vi "Game Mech.vi"() -> ()   [LabVIEW 2014]
uses:
  <vilib>/Rock Robotics/WPI/Solenoid/WPI_SolenoidValue.ctl
  <vilib>/Rock Robotics/WPI/Joystick/WPI_JoystickGetSetRefNum.vi
  <vilib>/Rock Robotics/Network Tables/SD Write Boolean Array.vi
  <vilib>/Rock Robotics/Network Tables/SD Write Numeric Array.vi
  <vilib>/Rock Robotics/WPI/Solenoid/WPI_SolenoidSetEnum.vi
  <vilib>/Rock Robotics/Network Tables/SD Write Number.vi
  <vilib>/addons/control/pid/NI_PID_pid.lvlib
  <vilib>/addons/control/pid/pid.llb/PID (DBL).vi
panel:
  in  "Controlling Mech":enum16{"Arm", "Left 2CAN", "Right 2CAN"}(ring)
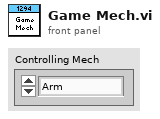
[diagram p1: front panel]
types:
  T1 = typedef "WPI_JoystickDevRef.ctl" = cluster{"Device":T2}
  T2 = typedef "WPI_JoystickDeviceEnum.ctl" = enum16{"USB 0", "USB 1", "USB 2", "USB 3", "USB 4", "USB 5"}
  T3 = cluster{"proportional gain (Kc)":dbl, "integral time (Ti, min)":dbl, "derivative time (Td, min)":dbl}
  T4 = typedef "WPI_PotentiometerDevRef.ctl" = cluster{"DevStatus":errorcluster, "Controller":T5, "Analog Channel":T6, "Invert Output":bool}
  T5 = typedef "FPGA_TypedefAnalogModule.ctl" = enum16{"Controller 1"}
  T6 = typedef "FPGA_AIChannel.ctl" = enum8{"AI 0", "AI 1", "AI 2", "AI 3", "AI MXP 0", "AI MXP 1", "AI MXP 2", "AI MXP 3", "Invalid"}
  T7 = typedef "WPI_SolenoidValue.ctl" = enum16{"Off", "On", "Forward", "Reverse"}
  T8 = typedef "WPI_SolenoidDevRef.ctl" = cluster{"DevStatus":errorcluster, "Pneumatics Control Module":u8, "Forward Solenoid Channel":T9, "Reverse Solenoid Channel":T9}
  T9 = typedef "WPI_SolenoidChannel.ctl" = enum8{"Solenoid 0", "Solenoid 1", "Solenoid 2", "Solenoid 3", "Solenoid 4", "Solenoid 5", "Solenoid 6", "Solenoid 7", "Invalid"}
  T10 = typedef "WPI_MotorControlDeviceRef.ctl" = cluster{"DeviceStatus":errorcluster, "Type":T11, "PWM":cluster{"Controller":T12, "PWM Channel":T13, "DeadBand":T14}, "CAN":cluster{"Device Number":u8, "Control Mode":T15, "Semaphore":T16, "Max Vout":dbl, "TalonSRX Control Mode":T17}, "Invert":bool, "TransformRef":T18, "InvTransformRef":T18}
  T11 = typedef "WPI_MotorControlType.ctl" = enum16{"PWM", "CAN", "CANTalonSRX"}
  T12 = typedef "FPGA_TypedefDigitalModule.ctl" = enum16{"Controller 1"}
  T13 = typedef "FPGA_DIOPWMChannel.ctl" = enum8{"PWM 0", "PWM 1", "PWM 2", "PWM 3", "PWM 4", "PWM 5", "PWM 6", "PWM 7", "PWM 8", "PWM 9", "PWM MXP 0", "PWM MXP 1", "PWM MXP 2", "PWM MXP 3", "PWM MXP 4", "PWM MXP 5", "PWM MXP 6", "PWM MXP 7", "PWM MXP 8", "PWM MXP 9", "Invalid"}
  T14 = typedef "WPI_PWMDeadband.ctl" = cluster{"Name":string, "maxPositivePwm":i32, "minPositivePwm":i32, "centerPwm":i32, "maxNegativePwm":i32, "minNegativePwm":i32, "angularRange":u16}
  T15 = typedef "WPI_CANJaguar_ControlMode.ctl" = enum8{"Percent VBus", "Current", "Speed", "Position", "Voltage"}
  T16 = typedef "Semaphore RefNum" = refnum<k1>
  T17 = typedef "WPI_CANTalonSRX_APIControlMode.ctl" = enum8{"Percent VBus", "Speed", "Position", "Slave", "Unchanged / Invalid"}
  T18 = typedef "WPI_PWMTransform_ConPane.ctl" = refnum<vi>
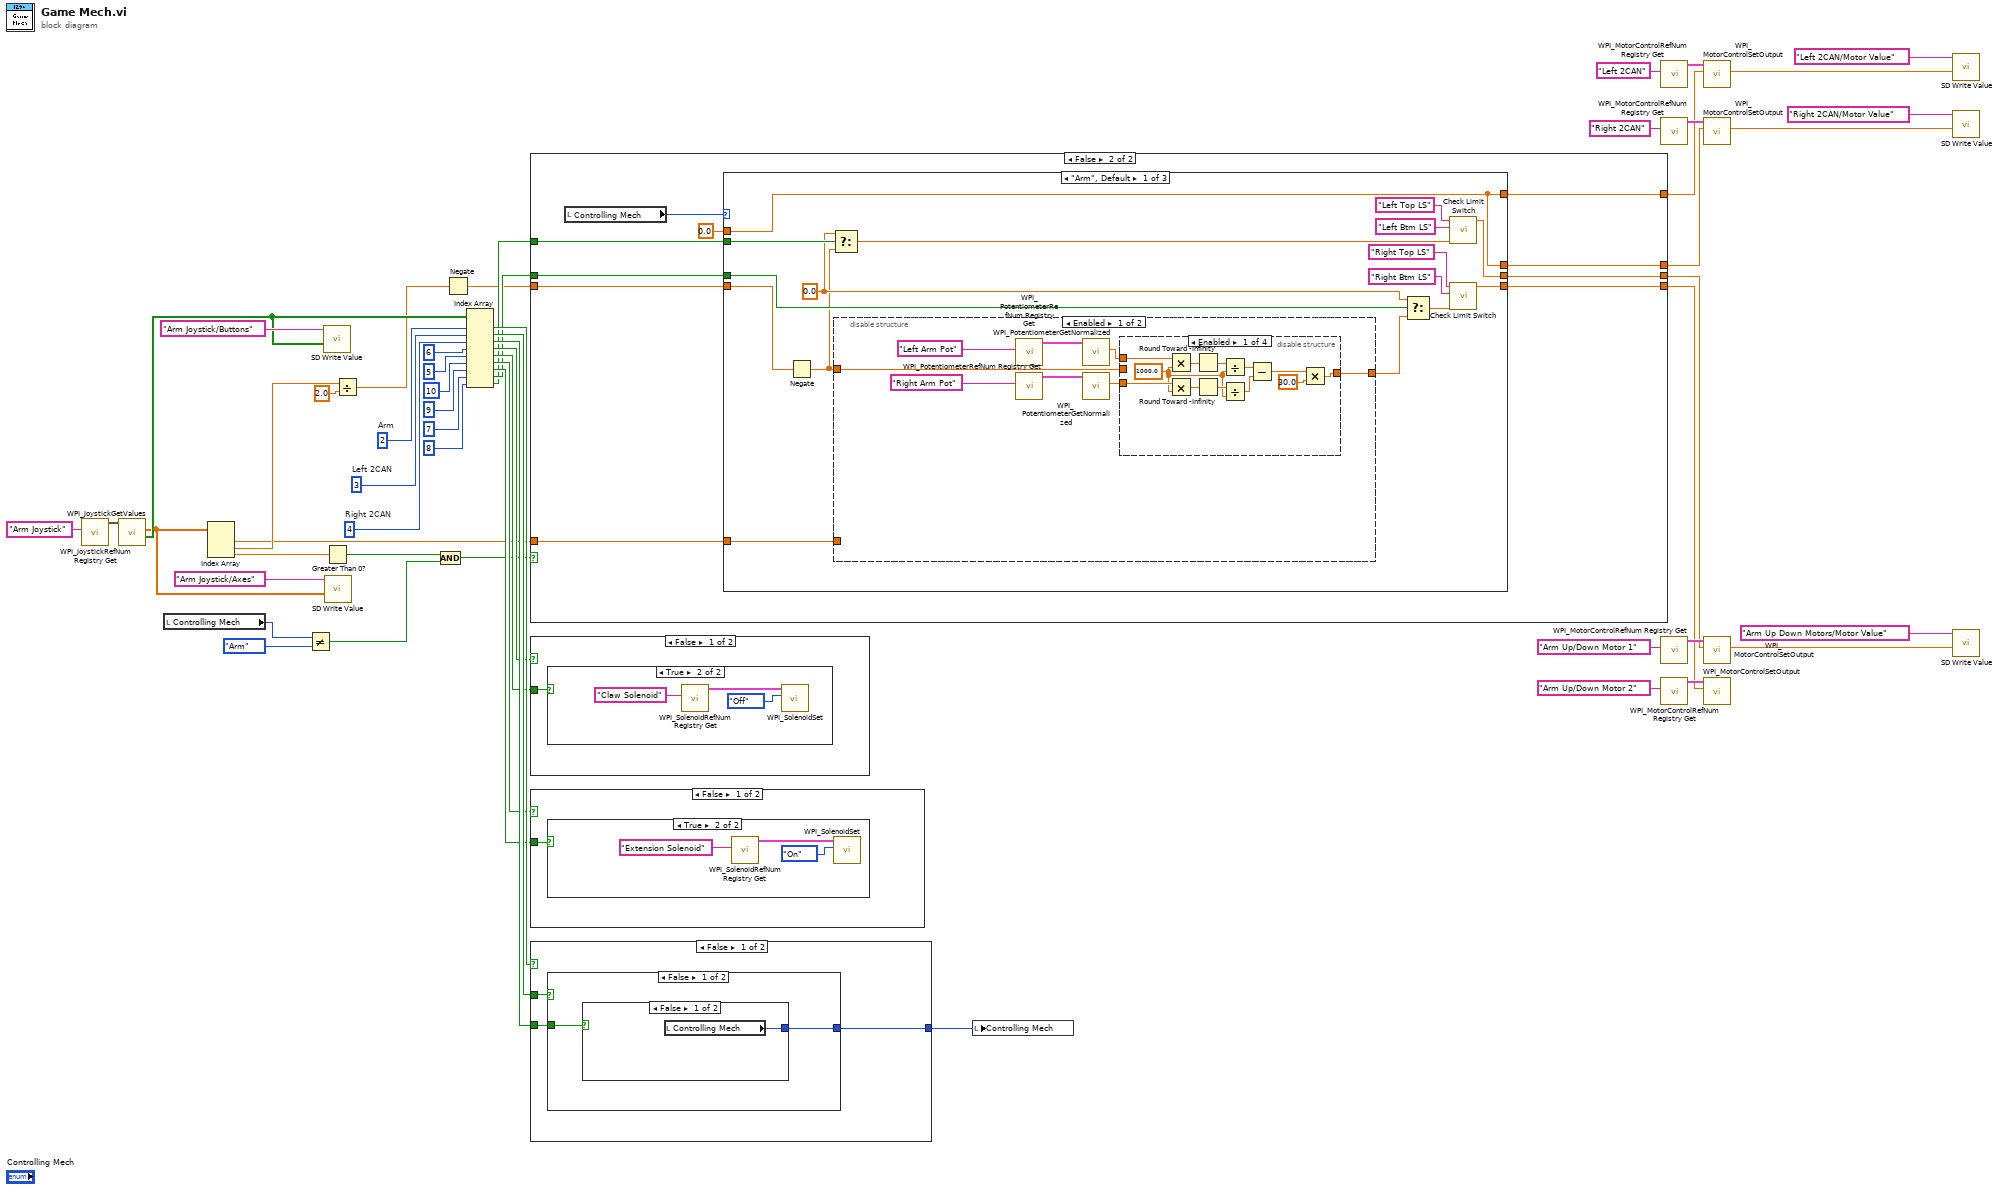
[diagram p0: block diagram]
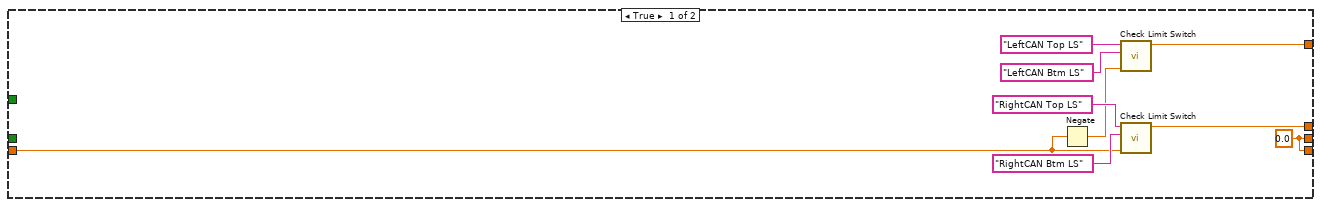
[diagram p2: hidden frame]
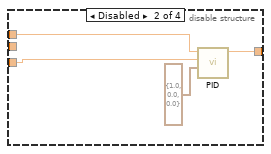
[diagram p3: hidden frame]
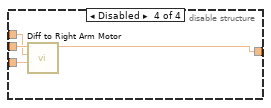
[diagram p5: hidden frame]
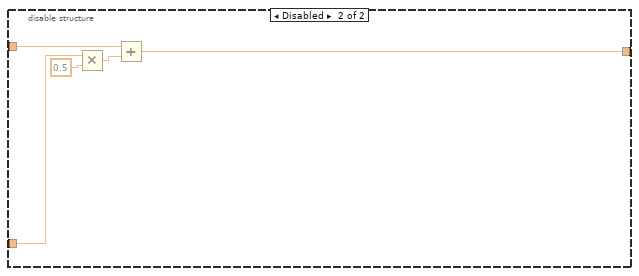
[diagram p6: hidden frame]
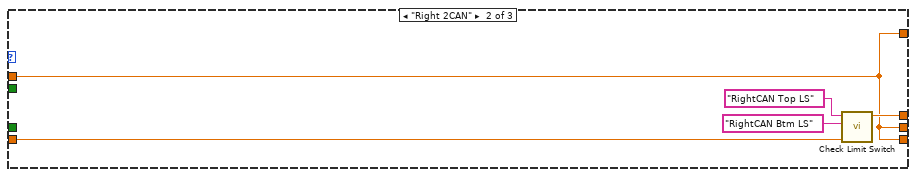
[diagram p7: hidden frame]
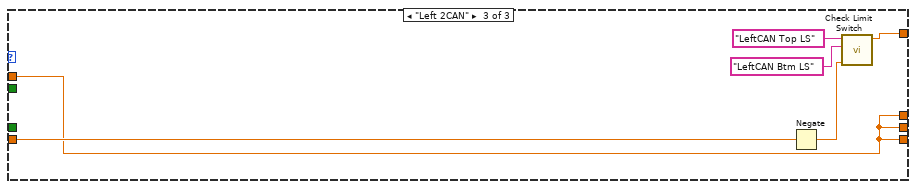
[diagram p8: hidden frame]
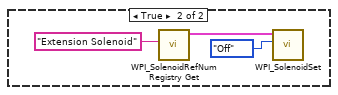
[diagram p10: hidden frame]
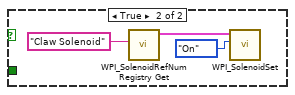
[diagram p12: hidden frame]
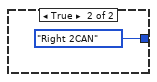
[diagram p13: hidden frame]
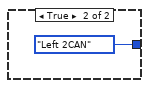
[diagram p14: hidden frame]
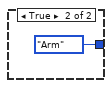
[diagram p15: hidden frame]
diagram:
  w30 = 4  # Right 2CAN
  w31 = 3  # Left 2CAN
  w32 = 2  # Arm
  n1 = call <vilib>:"WPI_JoystickRefNum Registry Get.vi"("refnum name"="Arm Joystick") -> ("JoystickDevRef"=w53:T1)  [unwired: 9 in, 1 out]
  n2 = call <vilib>:"WPI_JoystickGetValues.vi"("JoystickDevRef"=w53) -> ("Buttons"=w50:bool[], "Axes"=w49:dbl[])  [unwired: 6 in, 3 out]
  n3 = local read "Controlling Mech"() -> (w6:enum16{"Arm", "Left 2CAN", "Right 2CAN"})
  n4 = Index Array(array=w49) -> (element #1=w13:dbl, element #2=w14:dbl, element #3=w2:dbl)  [unwired: 3 in]
  n5 = Not Equal?(x=w6, y=enum16{"Arm", "Left 2CAN", "Right 2CAN"}."Arm" ("Controlling Mech")) -> (x != y?=w4:bool)
  n6 = call-poly <vilib>:"SD Write Value.vi"("Boolean Array"=w50, "Name"="Arm Joystick/Buttons") -> ()  [unwired: 8 in, 2 out]
  n7 = Greater Than 0?(x=w2) -> (x > 0?=w1:bool)
  n8 = call-poly <vilib>:"SD Write Value.vi"("Numeric Array"=w49, "Name"="Arm Joystick/Axes") -> ()  [unwired: 8 in, 2 out]
  n9 = Divide(x=w14, y=2.0) -> (x/y=w8:dbl)
  n10 = And(x=w1, y=w4) -> (x .and. y?=w3:bool)
  n11 = Negate(x=w8) -> (-x=w7:dbl)
  n12 = Index Array(array=w50, index #1=w32, index #2=w31, index #3=w30, index #4=6 ("index"), index #5=5 ("index"), index #6=10 ("index"), index #7=9 ("index"), index #8=7 ("index"), index #9=8 ("index")) -> (element #1=w29:bool, element #2=w28:bool, element #3=w27:bool, element #4=w24:bool, element #5=w23:bool, element #6=w17:bool, element #7=w16:bool, element #8=w10:bool, element #9=w9:bool)
  n13 = case shown="False" w3 {
    tunnel: [w55 w71] -> w33
    tunnel: [w55 w70] -> w22
    tunnel: [w57 w69] -> w21
    tunnel: [w56 w68] -> w20
    tunnel: w13 -> [_ w67]
    tunnel: w10 -> [_ w66]
    tunnel: w9 -> [_ w65]
    tunnel: w7 -> [w58 w64]
    frame True {
      w55 = 0.0 ("Checked Output")
      n14 = Negate(x=w58) -> (-x=w61:dbl)
      n15 = call "Check Limit Switch.vi"("Input"=w61, "Bottom LS RefNum Name"="LeftCAN Btm LS" ("refnum name"), "Forwards LS RefNum Name"="LeftCAN Top LS" ("refnum name")) -> ("Checked Output"=w57:dbl)  [unwired: 8 in]
      n16 = call "Check Limit Switch.vi"("Input"=w58, "Bottom LS RefNum Name"="RightCAN Btm LS" ("refnum name"), "Forwards LS RefNum Name"="RightCAN Top LS" ("refnum name")) -> ("Checked Output"=w56:dbl)  [unwired: 8 in]
    }
    frame False {
      n17 = local read "Controlling Mech"() -> (w73:enum16{"Arm", "Left 2CAN", "Right 2CAN"})
      n18 = case shown="\"Arm\", Default" w73 {
        tunnel: 0.0 -> [w89 w123 w128]
        tunnel: [w84 w123 w128] -> w71
        tunnel: [w89 w125 w128] -> w68
        tunnel: [w89 w123 w131] -> w69
        tunnel: [w83 w123 w128] -> w70
        tunnel: w67 -> [w82 _ _]
        tunnel: w66 -> [w81 _ _]
        tunnel: w65 -> [w77 _ _]
        tunnel: w64 -> [w74 w124 w129]
        frame "Arm", Default {
          w76 = 0.0 ("f")
          n19 = Negate(x=w74) -> (-x=w75:dbl)
          n20 = Select(t=w76, s=w77, f=w75) -> (s? t:f=w78:dbl)
          n21 = disable-structure shown="Enabled" {
            disable-tunnel: [w91 w118] -> w79
            disable-tunnel: w75 -> [w90 w120]
            disable-tunnel: w82 -> [_ w122]
            frame Enabled {
              n22 = call <vilib>:"WPI_PotentiometerRefNum Registry Get.vi"("refnum name"="Left Arm Pot") -> ("PotDevRef"=w94:T4)  [unwired: 9 in, 1 out]
              n23 = call <vilib>:"WPI_PotentiometerRefNum Registry Get.vi"("refnum name"="Right Arm Pot") -> ("PotDevRef"=w95:T4)  [unwired: 9 in, 1 out]
              n24 = call <vilib>:"WPI_PotentiometerGetNormalized.vi"("PotDevRef"=w94) -> ("Normalized Value"=w96:dbl)  [unwired: 8 in, 2 out]
              n25 = call <vilib>:"WPI_PotentiometerGetNormalized.vi"("PotDevRef"=w95) -> ("Normalized Value"=w97:dbl)  [unwired: 8 in, 2 out]
              n26 = disable-structure shown="Enabled" {
                disable-tunnel: w96 -> [w109 w112 _ w116]
                disable-tunnel: w97 -> [w108 w113 _ w115]
                disable-tunnel: [w99 w110 _ w114] -> w91
                disable-tunnel: w90 -> [_ _ _ w117]
                frame Enabled {
                  w101 = 1000.0
                  n27 = Multiply(x=w109, y=w101) -> (x*y=w107:dbl)
                  n28 = Multiply(x=w108, y=w101) -> (x*y=w106:dbl)
                  n29 = Round Toward -Infinity(1:w107) -> (0:w104:dbl)
                  n30 = Round Toward -Infinity(1:w106) -> (0:w105:dbl)
                  n31 = Divide(x=w104, y=w101) -> (x/y=w103:dbl)
                  n32 = Divide(x=w105, y=w101) -> (x/y=w102:dbl)
                  n33 = Subtract(x=w103, y=w102) -> (x-y=w100:dbl)
                  n34 = Multiply(x=w100, y=30.0) -> (x*y=w99:dbl)
                }
                frame Disabled {
                  n35 = call-poly <vilib>:"PID.vi"("PID gains"=T3 {"proportional gain (Kc)"=1.0, "integral time (Ti, min)"=0.0, "derivative time (Td, min)"=0.0}, "process variable"=w113, "setpoint"=w112) -> ("output"=w110:dbl)  [unwired: 7 in, 1 out]
                }
                frame Disabled {
                }
                frame Disabled {
                  n36 = call "Diff to Right Arm Motor.vi"("Right Pot"=w115, "Left Pot"=w116, "Joystick Axis"=w117) -> ("Right Arm Motor Axis"=w114:dbl)  [unwired: 8 in]
                }
              }
            }
            frame Disabled {
              n37 = Multiply(x=w122, y=0.5) -> (x*y=w119:dbl)
              n38 = Add(x=w120, y=w119) -> (x+y=w118:dbl)
            }
          }
          n39 = Select(t=w76, s=w81, f=w79) -> (s? t:f=w80:dbl)
          n40 = call "Check Limit Switch.vi"("Input"=w78, "Bottom LS RefNum Name"="Left Btm LS" ("refnum name"), "Forwards LS RefNum Name"="Left Top LS" ("refnum name")) -> ("Checked Output"=w84:dbl)  [unwired: 8 in]
          n41 = call "Check Limit Switch.vi"("Input"=w80, "Bottom LS RefNum Name"="Right Btm LS" ("refnum name"), "Forwards LS RefNum Name"="Right Top LS" ("refnum name")) -> ("Checked Output"=w83:dbl)  [unwired: 8 in]
        }
        frame "Right 2CAN" {
          n42 = call "Check Limit Switch.vi"("Input"=w124, "Bottom LS RefNum Name"="RightCAN Btm LS" ("refnum name"), "Forwards LS RefNum Name"="RightCAN Top LS" ("refnum name")) -> ("Checked Output"=w125:dbl)  [unwired: 8 in]
        }
        frame "Left 2CAN" {
          n43 = Negate(x=w129) -> (-x=w130:dbl)
          n44 = call "Check Limit Switch.vi"("Input"=w130, "Bottom LS RefNum Name"="LeftCAN Btm LS" ("refnum name"), "Forwards LS RefNum Name"="LeftCAN Top LS" ("refnum name")) -> ("Checked Output"=w131:dbl)  [unwired: 8 in]
        }
      }
    }
  }
  n45 = case shown="False" w24 {
    tunnel: w23 -> [w134 _]
    frame False {
      n46 = case shown="True" w134 {
        frame False {
        }
        frame True {
          n47 = call <vilib>:"WPI_SolenoidRefNum Registry Get.vi"("refnum name"="Claw Solenoid") -> ("SolenoidDevRef"=w137:T8)  [unwired: 9 in, 1 out]
          n48 = call-poly <vilib>:"WPI_SolenoidSet.vi"("Value"=WPI_SolenoidValue."Off" ("Arm Open?"), "SolenoidDevRef"=w137) -> ()  [unwired: 8 in, 2 out]
        }
      }
    }
    frame True {
      n49 = call <vilib>:"WPI_SolenoidRefNum Registry Get.vi"("refnum name"="Claw Solenoid") -> ("SolenoidDevRef"=w139:T8)  [unwired: 9 in, 1 out]
      n50 = call-poly <vilib>:"WPI_SolenoidSet.vi"("Value"=WPI_SolenoidValue."On" ("Arm Open?"), "SolenoidDevRef"=w139) -> ()  [unwired: 8 in, 2 out]
    }
  }
  n51 = case shown="False" w17 {
    tunnel: w16 -> [w141 _]
    frame False {
      n52 = case shown="True" w141 {
        frame False {
        }
        frame True {
          n53 = call <vilib>:"WPI_SolenoidRefNum Registry Get.vi"("refnum name"="Extension Solenoid") -> ("SolenoidDevRef"=w143:T8)  [unwired: 9 in, 1 out]
          n54 = call-poly <vilib>:"WPI_SolenoidSet.vi"("Value"=WPI_SolenoidValue."On" ("Arm Open?"), "SolenoidDevRef"=w143) -> ()  [unwired: 8 in, 2 out]
        }
      }
    }
    frame True {
      n55 = call <vilib>:"WPI_SolenoidRefNum Registry Get.vi"("refnum name"="Extension Solenoid") -> ("SolenoidDevRef"=w146:T8)  [unwired: 9 in, 1 out]
      n56 = call-poly <vilib>:"WPI_SolenoidSet.vi"("Value"=WPI_SolenoidValue."Off" ("Arm Open?"), "SolenoidDevRef"=w146) -> ()  [unwired: 8 in, 2 out]
    }
  }
  n57 = case shown="False" w29 {
    tunnel: [w150 enum16{"Arm", "Left 2CAN", "Right 2CAN"}."Arm" ("Controlling Mech")] -> w15
    tunnel: w28 -> [w149 _]
    tunnel: w27 -> [w148 _]
    frame False {
      n58 = case shown="False" w149 {
        tunnel: [w152 enum16{"Arm", "Left 2CAN", "Right 2CAN"}."Left 2CAN" ("Controlling Mech")] -> w150
        tunnel: w148 -> [w151 _]
        frame False {
          n59 = case shown="False" w151 {
            tunnel: [w153 enum16{"Arm", "Left 2CAN", "Right 2CAN"}."Right 2CAN" ("Controlling Mech")] -> w152
            frame False {
              n60 = local read "Controlling Mech"() -> (w153:enum16{"Arm", "Left 2CAN", "Right 2CAN"})
            }
            frame True {
            }
          }
        }
        frame True {
        }
      }
    }
    frame True {
    }
  }
  n61 = local write "Controlling Mech"(w15) -> ()
  n62 = call <vilib>:"WPI_MotorControlRefNum Registry Get.vi"("refnum name"="Left 2CAN") -> ("MotorControlDevRef"=w47:T10)  [unwired: 9 in, 1 out]
  n63 = call <vilib>:"WPI_MotorControlRefNum Registry Get.vi"("refnum name"="Right 2CAN") -> ("MotorControlDevRef"=w38:T10)  [unwired: 9 in, 1 out]
  n64 = call <vilib>:"WPI_MotorControlRefNum Registry Get.vi"("refnum name"="Arm Up/Down Motor 1") -> ("MotorControlDevRef"=w39:T10)  [unwired: 9 in, 1 out]
  n65 = call <vilib>:"WPI_MotorControlRefNum Registry Get.vi"("refnum name"="Arm Up/Down Motor 2") -> ("MotorControlDevRef"=w34:T10)  [unwired: 9 in, 1 out]
  n66 = call <vilib>:"WPI_MotorControlSetOutput.vi"("Output"=w21, "MotorControlDevRef"=w47) -> ("Motor Output"=w48:dbl)  [unwired: 7 in, 2 out]
  n67 = call <vilib>:"WPI_MotorControlSetOutput.vi"("Output"=w20, "MotorControlDevRef"=w38) -> ("Motor Output"=w45:dbl)  [unwired: 7 in, 2 out]
  n68 = call <vilib>:"WPI_MotorControlSetOutput.vi"("Output"=w33, "MotorControlDevRef"=w39) -> ("Motor Output"=w44:dbl)  [unwired: 7 in, 2 out]
  n69 = call <vilib>:"WPI_MotorControlSetOutput.vi"("Output"=w22, "MotorControlDevRef"=w34) -> ()  [unwired: 7 in, 3 out]
  n70 = call-poly <vilib>:"SD Write Value.vi"("Numeric"=w48, "Name"="Left 2CAN/Motor Value") -> ()  [unwired: 8 in, 2 out]
  n71 = call-poly <vilib>:"SD Write Value.vi"("Numeric"=w45, "Name"="Right 2CAN/Motor Value") -> ()  [unwired: 8 in, 2 out]
  n72 = call-poly <vilib>:"SD Write Value.vi"("Numeric"=w44, "Name"="Arm Up Down Motors/Motor Value") -> ()  [unwired: 8 in, 2 out]
